vi "ziExample-Scope.vi"() -> ()   [LabVIEW 2009]
doc: "Control a Zurich instrument device via the LabOne Labview API. \nRequirements: Zurich Instruments MFLI, HF2 or UHFLI \nThis example retrieves scope data from a Zurich Instruments instrument.\n\n© Zurich Instruments AG, www.zhinst.com"
uses:
  <instrlib>/Zurich Instruments LabOne/Public/Data/ziTypeScopeWave.ctl
  <instrlib>/Zurich Instruments LabOne/Public/Configure/ziSetValueDouble.vi
  <instrlib>/Zurich Instruments LabOne/Public/Data/ziGetEventScopeWave.vi
  <instrlib>/Zurich Instruments LabOne/Zurich Instruments LabOne.lvlib
  <vilib>/Analysis/NI_AALPro.lvlib
panel:
  out "Error Out":errorcluster
  in  "Address":string="DEV"
  out "FFT":T1(graph)
  out "ScopeWave":T2={"Timestamp (ticks)"=0, "Timestamp Trigger (ticks)"=0, "dt (s)"=0.0, "Channel Enable"=[], "Channel Input"=[], "Trigger Enable"=0, "Trigger Input"=0, "Channel BW Limit"=[], "Channel Math"=[], "Channel Scaling"=[], "Sequence Number"=0, "Segment Number"=0, "Block Number"=0, "Data Transfer Mode"=enum."Single Transfer", "Block Marker"=enum."None", "Flags"=0, "Sample Format"=enum."Float32 Interleaved", "Sample Count"=0, "Channel Offset"=[], "Data Int16"=[], "Data Int32"=[], "Data Float"=[]} {"dt (s)" format="%#_6p"}
  out "Selected Device":string
  out "Waveform":cluster{"dt (?)":dbl, "dt (s)":dbl, dbl[][]}(graph)
  in  "stop":bool
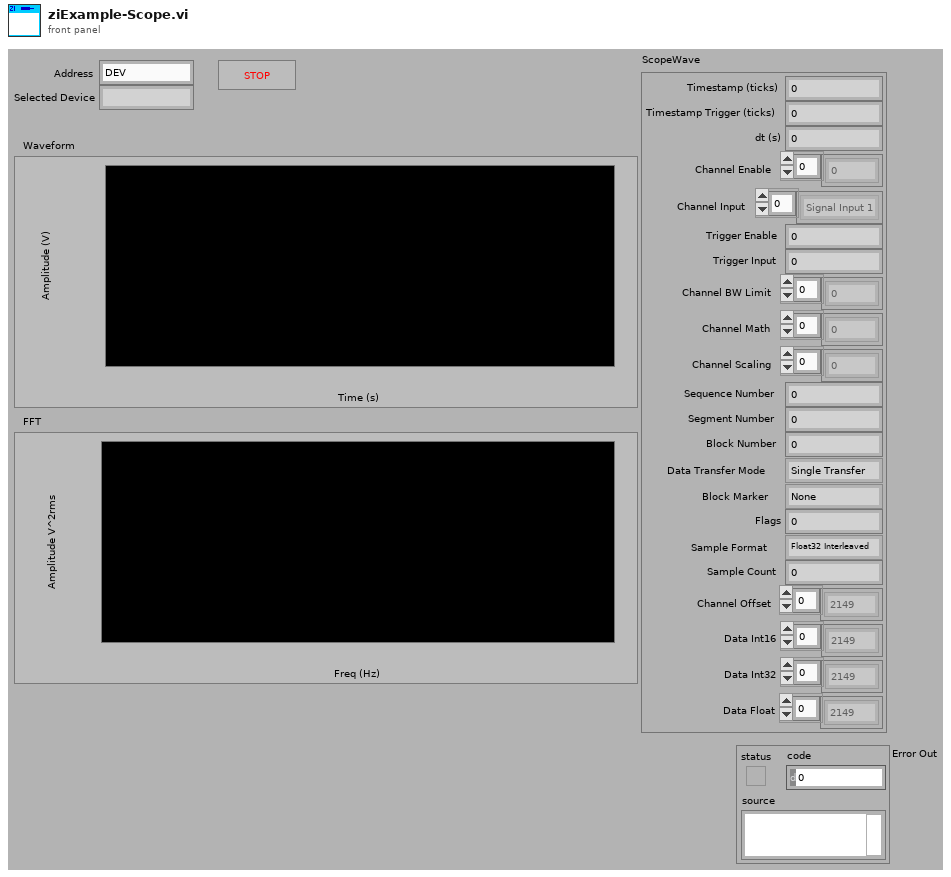
[diagram p1: front panel]
types:
  T1 = cluster{"dt (?)":dbl, "df":dbl, "Power Spectrum (V^2 rms)":dbl[][]}
  T2 = typedef "Zurich Instruments LabOne.lvlib/ziTypeScopeWave.ctl" = cluster{"Timestamp (ticks)":u64, "Timestamp Trigger (ticks)":u64, "dt (s)":dbl, "Channel Enable":u8[], "Channel Input":enum8{"Signal Input 1", "Signal Input 2", "Trigger Input 1", "Trigger Input 2", "Aux Output 1", "Aux Output 2", "Aux Output 3", "Aux Output 4", "Aux Input 1", "Aux Input 2"}[], "Trigger Enable":u64, "Trigger Input":u64, "Channel BW Limit":u8[], "Channel Math":u8[], "Channel Scaling":sgl[], "Sequence Number":u32, "Segment Number":u32, "Block Number":u32, "Data Transfer Mode":enum8{"Single Transfer", "Block Transfer", "Continuous Transfer", "FFT Single Transfer"}, "Block Marker":enum8{"None", "End of Block"}, "Flags":u8, "Sample Format":enum8{"Int16", "Int32", "Float32", "reserved", "Int16 Interleaved", "Int32 Interleaved", "Float32 Interleaved"}, "Sample Count":u32, "Channel Offset":dbl[], "Data Int16":i16[], "Data Int32":i32[], "Data Float":sgl[]}
  T3 = typedef "Zurich Instruments LabOne.lvlib/ziTypeHandle.ctl" = cluster{"handleValid":bool, "Conn":u64, "Path Prefix":string, "Handle":u64, "Connected":bool, "Clockbase(s)":dbl}
  T4 = enum8{"Int16", "Int32", "Float32", "reserved", "Int16 Interleaved", "Int32 Interleaved", "Float32 Interleaved"}
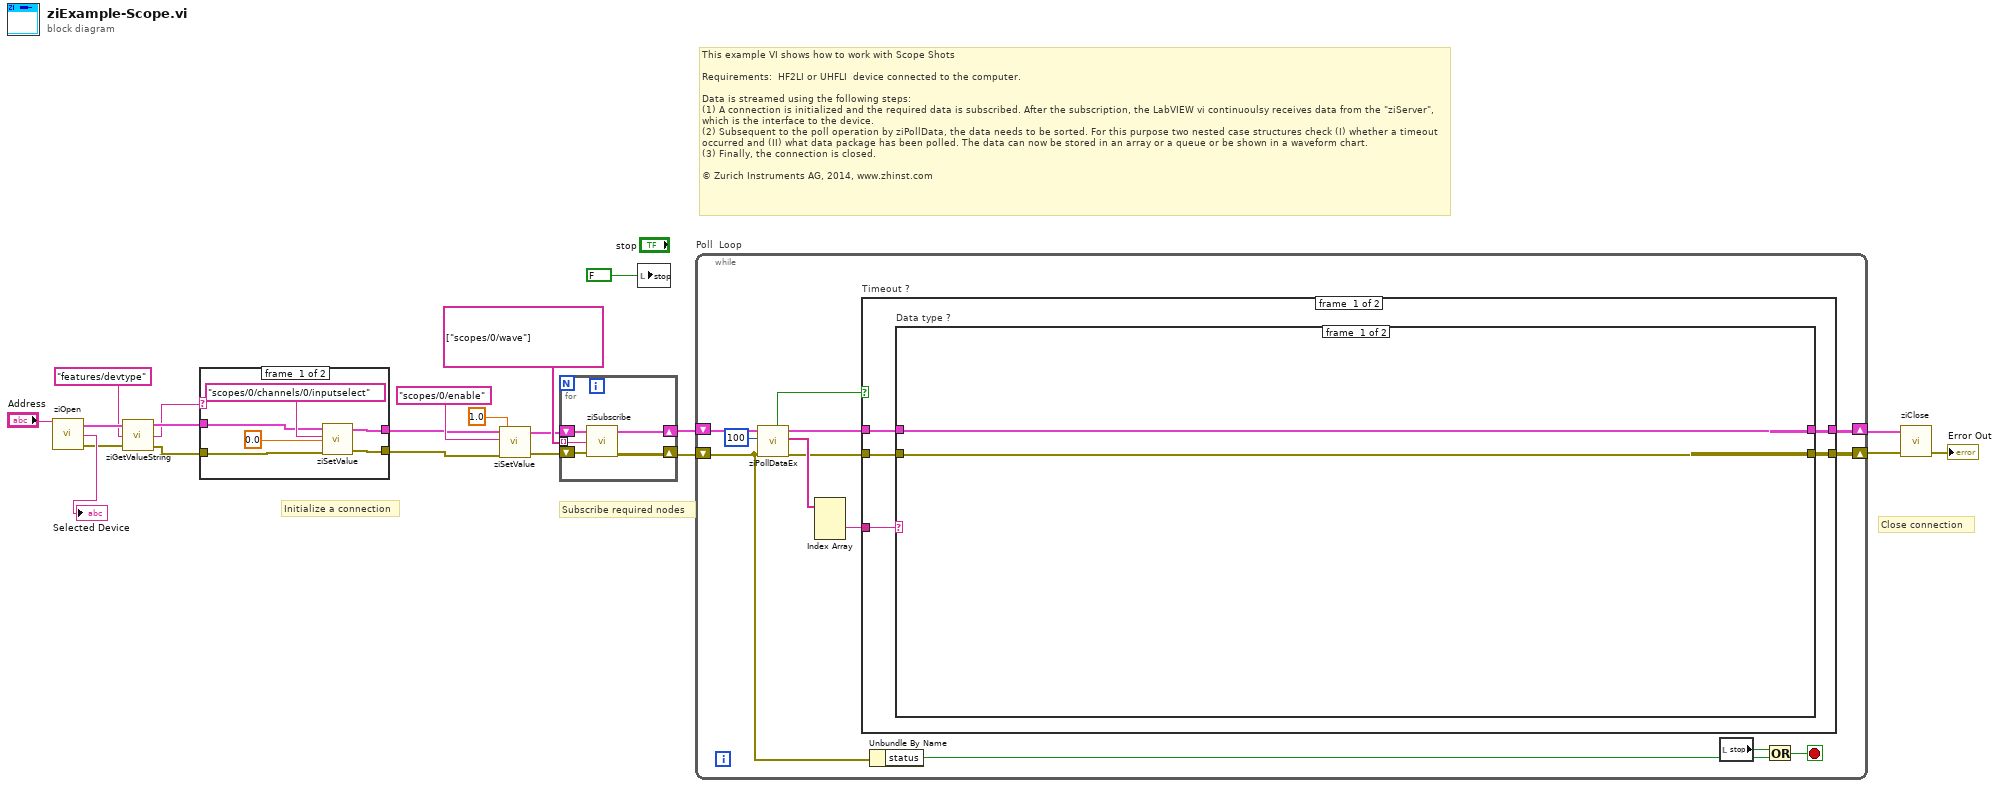
[diagram p0: block diagram]
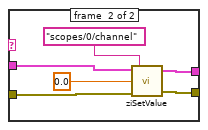
[diagram p2: hidden frame]
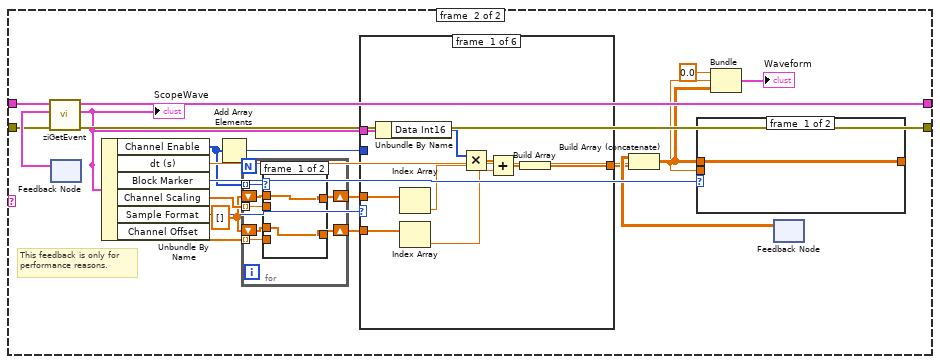
[diagram p3: hidden frame]
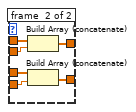
[diagram p4: hidden frame]
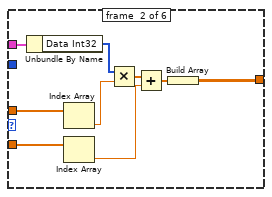
[diagram p5: hidden frame]
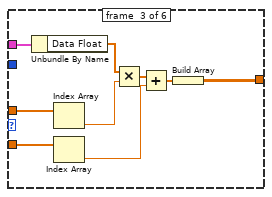
[diagram p6: hidden frame]
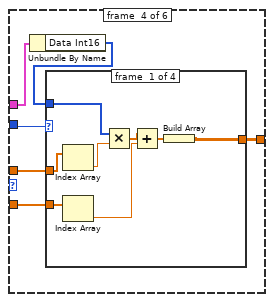
[diagram p7: hidden frame]
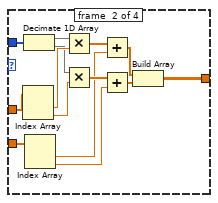
[diagram p8: hidden frame]
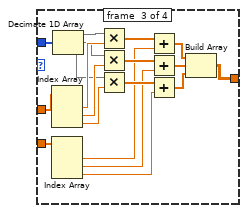
[diagram p9: hidden frame]
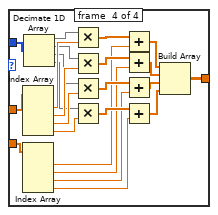
[diagram p10: hidden frame]
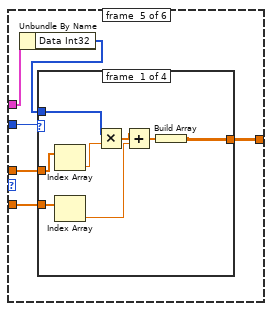
[diagram p11: hidden frame]
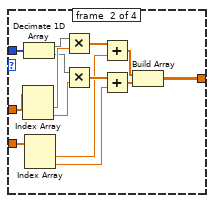
[diagram p12: hidden frame]
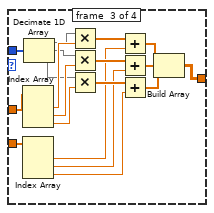
[diagram p13: hidden frame]
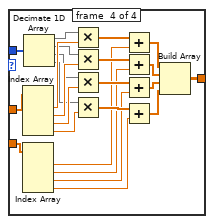
[diagram p14: hidden frame]
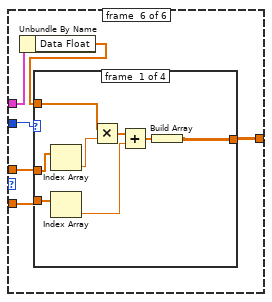
[diagram p15: hidden frame]
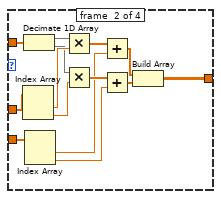
[diagram p16: hidden frame]
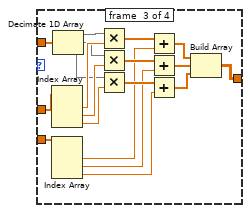
[diagram p17: hidden frame]
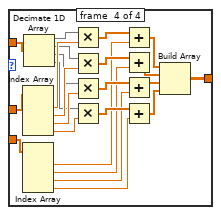
[diagram p18: hidden frame]
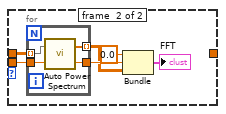
[diagram p19: hidden frame]
diagram:
  # "Close connection"
  # "Initialize a connection"
  # "Subscribe required nodes"
  # "This example VI shows how to work with Scope Shots\n\nRequirements:  HF2LI or UHFLI  device connected to the computer.\n\nData is streamed using the following steps:\n(1) A connection is initialized and the required data is subscribed. After the subscription, the LabVIEW vi continuoulsy receives data from the \"ziServer\", which is the interface to the device. \n(2) Subsequent to the poll operation by ziPollData, the data needs to be sorted. For this purpose two nested case structures check (I) whether a timeout occurred and (II) what data package has been polled. The data can now be stored in an array or a queue or be shown in a waveform chart. \n(3) Finally, the connection is closed. \n\n© Zurich Instruments AG, 2014, www.zhinst.com"
  n1 = call <instrlib>:"ziOpen.vi"("Address"="Address") -> ("Error Out"=w6:errorcluster, "Selected Device"=→"Selected Device":string, "HandleOut"=w3:T3)  [unwired: 1 in, 2 out]
  n2 = call <instrlib>:"ziGetValueString.vi"("error in"=w6, "Path"="features/devtype", "Handle In"=w3) -> ("error out"=w5:errorcluster, "Value"=w2:string, "Handle Out"=w4:T3)
  n3 = case shown="\"HF2IS\", \"HF2LI\"" w2 {
    tunnel: w4 -> [w25 w31]
    tunnel: w5 -> [w24 w30]
    tunnel: [w23 w29] -> w8
    tunnel: [w22 w28] -> w7
    frame #0 {
      n4 = call-poly <instrlib>:"ziSetValue.vi"("Error In"=w24, "Value"=0.0, "Path"="scopes/0/channels/0/inputselect", "Handle In"=w25) -> ("Error Out"=w23:errorcluster, "Handle Out"=w22:T3)  [unwired: 1 in]
    }
    frame #1 {
      n5 = call-poly <instrlib>:"ziSetValue.vi"("Error In"=w30, "Value"=0.0, "Path"="scopes/0/channel", "Handle In"=w31) -> ("Error Out"=w29:errorcluster, "Handle Out"=w28:T3)  [unwired: 1 in]
    }
  }
  n6 = call-poly <instrlib>:"ziSetValue.vi"("Error In"=w8, "Value"=1.0, "Path"="scopes/0/enable", "Handle In"=w7) -> ("Error Out"=w12:errorcluster, "Handle Out"=w13:T3)  [unwired: 1 in]
  n7 = for {
    shift-right: [w38] -> w17
    shift-left: w13 -> [w36]
    shift-right: [w37] -> w16
    shift-left: w12 -> [w35]
    tunnel: string[] ["scopes/0/wave"] -> [w34] mode=indexing
    n8 = call <instrlib>:"ziSubscribe.vi"("error in"=w35, "Path ()"=w34, "Handle In"=w36) -> ("error out"=w37:errorcluster, "Handle Out"=w38:T3)  [unwired: 1 in]
  }
  n9 = local write "stop"(FALSE ("Record")) -> ()
  n10 = while "Poll  Loop" {
    shift-right: [w45] -> w18
    shift-left: w17 -> [w51]
    shift-right: [w43] -> w19
    shift-left: w16 -> [w42]
    stop <- w39 stop-if-true
    n11 = call <instrlib>:"ziPollDataEx.vi"("error in"=w42, "Timeout ms (50)"=100 ("TimeOut ms (50)"), "Handle In"=w51) -> ("error out"=w44:errorcluster, "PathArray"=w48:string[], "Handle Out"=w46:T3, "Timed Out"=w49:bool)  [unwired: 1 in, 4 out]
    n12 = Index Array(array=w48) -> (element #2=w47:string)  [unwired: 3 in, 2 out]
    n13 = case "Timeout ?" shown="False" w49 {
      tunnel: w47 -> [w56 _]
      tunnel: w46 -> [w55 w348]
      tunnel: [w54 w348] -> w45
      tunnel: w44 -> [w53 w347]
      tunnel: [w52 w347] -> w43
      frame #0 {
        n14 = case "Data type ?" shown="\"SCOPES\"" w56 {
          tunnel: w55 -> [w58 w80]
          tunnel: [w58 w79] -> w54
          tunnel: w53 -> [w57 w75]
          tunnel: [w57 w74] -> w52
          frame #0 {
          }
          frame #1 {
            w59 = dbl[] []
            # "This feedback is only for\nperformance reasons."
            n15 = feedback #1() -> (w78:T2)  [unwired: 1 in]
            n16 = call-poly <instrlib>:"ziGetEvent.vi"("Error In"=w75, "ScopeWave In"=w78, "Handle In"=w80) -> ("Error Out"=w74:errorcluster, "ScopeWave Out"=w67:T2, "Handle Out"=w79:T3)  [unwired: 6 in]
            "ScopeWave" <- w67
            n17 = Unbundle By Name(w67) -> ("Channel Enable"=w64:u8[], "dt (s)"=w69:dbl, "Block Marker"=w73:enum8{"None", "End of Block"}, "Channel Scaling"=w63:sgl[], "Sample Format"=w68:T4, "Channel Offset"=w61:dbl[])
            n18 = Add Array Elements(numeric array=w64) -> (sum=w65:u8)
            n19 = for {
              tunnel: w63 -> [w87] mode=indexing
              tunnel: w64 -> [w84] mode=indexing
              shift-right: [w85] -> w62
              shift-left: w59 -> [w86]
              tunnel: w61 -> [w83] mode=indexing
              shift-right: [w82] -> w60
              shift-left: w59 -> [w81]
              n20 = case shown="1" w84 {
                tunnel: w87 -> [_ w95]
                tunnel: w86 -> [w89 w94]
                tunnel: [w89 w93] -> w85
                tunnel: w83 -> [_ w92]
                tunnel: [w88 w91] -> w82
                tunnel: w81 -> [w88 w90]
                frame #0 {
                }
                frame #1 {
                  n21 = Build Array (concatenate)(w94, w95) -> (w93:dbl[])
                  n22 = Build Array (concatenate)(w90, w92) -> (w91:dbl[])
                }
              }
            }
            n23 = case shown="\"Int32 Interleaved\"" w68 {
              tunnel: w62 -> [w104 w108 w117 w126 w196 w267]
              tunnel: [w100 w105 w115 w125 w198 w269] -> w66
              tunnel: w67 -> [w102 w113 w122 w128 w199 w270]
              tunnel: w65 -> [_ _ _ w124 w194 w266]
              tunnel: w60 -> [w99 w107 w116 w123 w197 w268]
              frame #0 {
                n24 = Unbundle By Name(w102) -> ("Data Int16"=w101:i16[])
                n25 = Index Array(array=w104) -> (element=w103:dbl)  [unwired: 1 in]
                n26 = Index Array(array=w99) -> (element=w96:dbl)  [unwired: 1 in]
                n27 = Multiply(x=w101, y=w103) -> (x*y=w98:dbl[])
                n28 = Add(x=w98, y=w96) -> (x+y=w97:dbl[])
                n29 = Build Array(w97) -> (w100:dbl[][])
              }
              frame #1 {
                n30 = Unbundle By Name(w113) -> ("Data Int32"=w106:i32[])
                n31 = Index Array(array=w108) -> (element=w112:dbl)  [unwired: 1 in]
                n32 = Index Array(array=w107) -> (element=w109:dbl)  [unwired: 1 in]
                n33 = Multiply(x=w106, y=w112) -> (x*y=w111:dbl[])
                n34 = Add(x=w111, y=w109) -> (x+y=w110:dbl[])
                n35 = Build Array(w110) -> (w105:dbl[][])
              }
              frame #2 {
                n36 = Unbundle By Name(w122) -> ("Data Float"=w114:sgl[])
                n37 = Index Array(array=w117) -> (element=w121:dbl)  [unwired: 1 in]
                n38 = Index Array(array=w116) -> (element=w118:dbl)  [unwired: 1 in]
                n39 = Multiply(x=w114, y=w121) -> (x*y=w120:dbl[])
                n40 = Add(x=w120, y=w118) -> (x+y=w119:dbl[])
                n41 = Build Array(w119) -> (w115:dbl[][])
              }
              frame #3 {
                n42 = Unbundle By Name(w128) -> ("Data Int16"=w127:i16[])
                n43 = case shown="4" w124 {
                  tunnel: w127 -> [w135 w150 w169 w193]
                  tunnel: [w136 w149 w168 w192] -> w125
                  tunnel: w126 -> [w134 w148 w167 w191]
                  tunnel: w123 -> [w130 w137 w153 w174]
                  frame #0 {
                    n44 = Index Array(array=w134) -> (element=w133:dbl)  [unwired: 1 in]
                    n45 = Index Array(array=w130) -> (element=w129:dbl)  [unwired: 1 in]
                    n46 = Multiply(x=w135, y=w133) -> (x*y=w131:dbl[])
                    n47 = Add(x=w131, y=w129) -> (x+y=w132:dbl[])
                    n48 = Build Array(w132) -> (w136:dbl[][])
                  }
                  frame #1 {
                    n49 = Index Array(array=w148) -> (element #1=w147:dbl, element #2=w144:dbl)  [unwired: 2 in]
                    n50 = Decimate 1D Array(w150) -> (w146:i16[], w145:i16[])
                    n51 = Index Array(array=w137) -> (element #1=w138:dbl, element #2=w139:dbl)  [unwired: 2 in]
                    n52 = Multiply(x=w146, y=w147) -> (x*y=w142:dbl[])
                    n53 = Multiply(x=w145, y=w144) -> (x*y=w141:dbl[])
                    n54 = Add(x=w142, y=w138) -> (x+y=w143:dbl[])
                    n55 = Add(x=w141, y=w139) -> (x+y=w140:dbl[])
                    n56 = Build Array(w143, w140) -> (w149:dbl[][])
                  }
                  frame #2 {
                    n57 = Index Array(array=w167) -> (element #1=w166:dbl, element #2=w163:dbl, element #3=w162:dbl)  [unwired: 3 in]
                    n58 = Index Array(array=w153) -> (element #1=w156:dbl, element #2=w155:dbl, element #3=w154:dbl)  [unwired: 3 in]
                    n59 = Decimate 1D Array(w169) -> (w165:i16[], w164:i16[], w161:i16[])
                    n60 = Multiply(x=w165, y=w166) -> (x*y=w157:dbl[])
                    n61 = Multiply(x=w164, y=w163) -> (x*y=w158:dbl[])
                    n62 = Multiply(x=w161, y=w162) -> (x*y=w159:dbl[])
                    n63 = Add(x=w157, y=w156) -> (x+y=w160:dbl[])
                    n64 = Add(x=w158, y=w155) -> (x+y=w152:dbl[])
                    n65 = Add(x=w159, y=w154) -> (x+y=w151:dbl[])
                    n66 = Build Array(w160, w152, w151) -> (w168:dbl[][])
                  }
                  frame #3 {
                    n67 = Index Array(array=w191) -> (element #1=w190:dbl, element #2=w187:dbl, element #3=w186:dbl, element #4=w184:dbl)  [unwired: 4 in]
                    n68 = Index Array(array=w174) -> (element #1=w173:dbl, element #2=w172:dbl, element #3=w171:dbl, element #4=w170:dbl)  [unwired: 4 in]
                    n69 = Decimate 1D Array(w193) -> (w189:i16[], w188:i16[], w185:i16[], w183:i16[])
                    n70 = Multiply(x=w189, y=w190) -> (x*y=w182:dbl[])
                    n71 = Multiply(x=w188, y=w187) -> (x*y=w181:dbl[])
                    n72 = Multiply(x=w185, y=w186) -> (x*y=w180:dbl[])
                    n73 = Multiply(x=w183, y=w184) -> (x*y=w179:dbl[])
                    n74 = Add(x=w182, y=w173) -> (x+y=w175:dbl[])
                    n75 = Add(x=w181, y=w172) -> (x+y=w176:dbl[])
                    n76 = Add(x=w180, y=w171) -> (x+y=w177:dbl[])
                    n77 = Add(x=w179, y=w170) -> (x+y=w178:dbl[])
                    n78 = Build Array(w175, w176, w177, w178) -> (w192:dbl[][])
                  }
                }
              }
              frame #4 {
                n79 = Unbundle By Name(w199) -> ("Data Int32"=w195:i32[])
                n80 = case shown="4" w194 {
                  tunnel: w195 -> [w206 w221 w240 w264]
                  tunnel: [w207 w220 w239 w263] -> w198
                  tunnel: w196 -> [w205 w219 w238 w262]
                  tunnel: w197 -> [w201 w208 w224 w245]
                  frame #0 {
                    n81 = Index Array(array=w205) -> (element=w204:dbl)  [unwired: 1 in]
                    n82 = Index Array(array=w201) -> (element=w200:dbl)  [unwired: 1 in]
                    n83 = Multiply(x=w206, y=w204) -> (x*y=w202:dbl[])
                    n84 = Add(x=w202, y=w200) -> (x+y=w203:dbl[])
                    n85 = Build Array(w203) -> (w207:dbl[][])
                  }
                  frame #1 {
                    n86 = Index Array(array=w219) -> (element #1=w218:dbl, element #2=w215:dbl)  [unwired: 2 in]
                    n87 = Decimate 1D Array(w221) -> (w217:i32[], w216:i32[])
                    n88 = Index Array(array=w208) -> (element #1=w209:dbl, element #2=w210:dbl)  [unwired: 2 in]
                    n89 = Multiply(x=w217, y=w218) -> (x*y=w213:dbl[])
                    n90 = Multiply(x=w216, y=w215) -> (x*y=w212:dbl[])
                    n91 = Add(x=w213, y=w209) -> (x+y=w214:dbl[])
                    n92 = Add(x=w212, y=w210) -> (x+y=w211:dbl[])
                    n93 = Build Array(w214, w211) -> (w220:dbl[][])
                  }
                  frame #2 {
                    n94 = Index Array(array=w238) -> (element #1=w237:dbl, element #2=w234:dbl, element #3=w233:dbl)  [unwired: 3 in]
                    n95 = Index Array(array=w224) -> (element #1=w227:dbl, element #2=w226:dbl, element #3=w225:dbl)  [unwired: 3 in]
                    n96 = Decimate 1D Array(w240) -> (w236:i32[], w235:i32[], w232:i32[])
                    n97 = Multiply(x=w236, y=w237) -> (x*y=w228:dbl[])
                    n98 = Multiply(x=w235, y=w234) -> (x*y=w229:dbl[])
                    n99 = Multiply(x=w232, y=w233) -> (x*y=w230:dbl[])
                    n100 = Add(x=w228, y=w227) -> (x+y=w231:dbl[])
                    n101 = Add(x=w229, y=w226) -> (x+y=w223:dbl[])
                    n102 = Add(x=w230, y=w225) -> (x+y=w222:dbl[])
                    n103 = Build Array(w231, w223, w222) -> (w239:dbl[][])
                  }
                  frame #3 {
                    n104 = Index Array(array=w262) -> (element #1=w261:dbl, element #2=w258:dbl, element #3=w257:dbl, element #4=w255:dbl)  [unwired: 4 in]
                    n105 = Index Array(array=w245) -> (element #1=w244:dbl, element #2=w243:dbl, element #3=w242:dbl, element #4=w241:dbl)  [unwired: 4 in]
                    n106 = Decimate 1D Array(w264) -> (w260:i32[], w259:i32[], w256:i32[], w254:i32[])
                    n107 = Multiply(x=w260, y=w261) -> (x*y=w253:dbl[])
                    n108 = Multiply(x=w259, y=w258) -> (x*y=w252:dbl[])
                    n109 = Multiply(x=w256, y=w257) -> (x*y=w251:dbl[])
                    n110 = Multiply(x=w254, y=w255) -> (x*y=w250:dbl[])
                    n111 = Add(x=w253, y=w244) -> (x+y=w246:dbl[])
                    n112 = Add(x=w252, y=w243) -> (x+y=w247:dbl[])
                    n113 = Add(x=w251, y=w242) -> (x+y=w248:dbl[])
                    n114 = Add(x=w250, y=w241) -> (x+y=w249:dbl[])
                    n115 = Build Array(w246, w247, w248, w249) -> (w263:dbl[][])
                  }
                }
              }
              frame #5 {
                n116 = Unbundle By Name(w270) -> ("Data Float"=w265:sgl[])
                n117 = case shown="4" w266 {
                  tunnel: w265 -> [w277 w292 w311 w335]
                  tunnel: [w278 w291 w310 w334] -> w269
                  tunnel: w267 -> [w276 w290 w309 w333]
                  tunnel: w268 -> [w272 w279 w295 w316]
                  frame #0 {
                    n118 = Index Array(array=w276) -> (element=w275:dbl)  [unwired: 1 in]
                    n119 = Index Array(array=w272) -> (element=w271:dbl)  [unwired: 1 in]
                    n120 = Multiply(x=w277, y=w275) -> (x*y=w273:dbl[])
                    n121 = Add(x=w273, y=w271) -> (x+y=w274:dbl[])
                    n122 = Build Array(w274) -> (w278:dbl[][])
                  }
                  frame #1 {
                    n123 = Index Array(array=w290) -> (element #1=w289:dbl, element #2=w286:dbl)  [unwired: 2 in]
                    n124 = Decimate 1D Array(w292) -> (w288:sgl[], w287:sgl[])
                    n125 = Index Array(array=w279) -> (element #1=w280:dbl, element #2=w281:dbl)  [unwired: 2 in]
                    n126 = Multiply(x=w288, y=w289) -> (x*y=w284:dbl[])
                    n127 = Multiply(x=w287, y=w286) -> (x*y=w283:dbl[])
                    n128 = Add(x=w284, y=w280) -> (x+y=w285:dbl[])
                    n129 = Add(x=w283, y=w281) -> (x+y=w282:dbl[])
                    n130 = Build Array(w285, w282) -> (w291:dbl[][])
                  }
                  frame #2 {
                    n131 = Index Array(array=w309) -> (element #1=w308:dbl, element #2=w305:dbl, element #3=w304:dbl)  [unwired: 3 in]
                    n132 = Index Array(array=w295) -> (element #1=w298:dbl, element #2=w297:dbl, element #3=w296:dbl)  [unwired: 3 in]
                    n133 = Decimate 1D Array(w311) -> (w307:sgl[], w306:sgl[], w303:sgl[])
                    n134 = Multiply(x=w307, y=w308) -> (x*y=w299:dbl[])
                    n135 = Multiply(x=w306, y=w305) -> (x*y=w300:dbl[])
                    n136 = Multiply(x=w303, y=w304) -> (x*y=w301:dbl[])
                    n137 = Add(x=w299, y=w298) -> (x+y=w302:dbl[])
                    n138 = Add(x=w300, y=w297) -> (x+y=w294:dbl[])
                    n139 = Add(x=w301, y=w296) -> (x+y=w293:dbl[])
                    n140 = Build Array(w302, w294, w293) -> (w310:dbl[][])
                  }
                  frame #3 {
                    n141 = Index Array(array=w333) -> (element #1=w332:dbl, element #2=w329:dbl, element #3=w328:dbl, element #4=w326:dbl)  [unwired: 4 in]
                    n142 = Index Array(array=w316) -> (element #1=w315:dbl, element #2=w314:dbl, element #3=w313:dbl, element #4=w312:dbl)  [unwired: 4 in]
                    n143 = Decimate 1D Array(w335) -> (w331:sgl[], w330:sgl[], w327:sgl[], w325:sgl[])
                    n144 = Multiply(x=w331, y=w332) -> (x*y=w324:dbl[])
                    n145 = Multiply(x=w330, y=w329) -> (x*y=w323:dbl[])
                    n146 = Multiply(x=w327, y=w328) -> (x*y=w322:dbl[])
                    n147 = Multiply(x=w325, y=w326) -> (x*y=w321:dbl[])
                    n148 = Add(x=w324, y=w315) -> (x+y=w317:dbl[])
                    n149 = Add(x=w323, y=w314) -> (x+y=w318:dbl[])
                    n150 = Add(x=w322, y=w313) -> (x+y=w319:dbl[])
                    n151 = Add(x=w321, y=w312) -> (x+y=w320:dbl[])
                    n152 = Build Array(w317, w318, w319, w320) -> (w334:dbl[][])
                  }
                }
              }
            }
            n153 = feedback #2() -> (w71:dbl[][])  [unwired: 1 in]
            n154 = Build Array (concatenate)(w71, w66) -> (w70:dbl[][])
            n155 = case shown="\"End of Block\"" w73 {
              tunnel: w70 -> [w336 w341]
              tunnel: [w336 _] -> w72
              tunnel: w69 -> [_ w342]
              frame #0 {
              }
              frame #1 {
                n156 = for {
                  tunnel: w342 -> [w346]
                  tunnel: w341 -> [w345] mode=indexing
                  tunnel: [w344] -> w338
                  tunnel: [w343] -> w337 mode=indexing
                  n157 = call <vilib>:"Auto Power Spectrum.vi"("dt"=w346, "Signal (V)"=w345) -> ("df"=w344:dbl, "Power Spectrum (V^2 rms)"=w343:dbl[])
                }
                n158 = Bundle("dt (?)"=0.0, "df"=w338, "Power Spectrum (V^2 rms)"=w337) -> (→"FFT":T1)  [unwired: 1 in]
              }
            }
            n159 = Bundle("dt (?)"=0.0, "dt (s)"=w69, w70) -> (→"Waveform":cluster{"dt (?)":dbl, "dt (s)":dbl, dbl[][]})  [unwired: 1 in]
          }
        }
      }
      frame #1 {
        # "Timeout, no action."
      }
    }
    n160 = Unbundle By Name(w42) -> ("status"=w41:bool)
    n161 = local read "stop"() -> (w40:bool)
    n162 = Or(x=w40, y=w41) -> (x .or. y?=w39:bool)
  }
  n163 = call <instrlib>:"ziClose.vi"("Error In"=w19, "Handle In"=w18) -> ("Error Out"=→"Error Out":errorcluster)  [unwired: 3 out]
